vi "Module Init.vi"(8 "error in (no error)":errorcluster, 11 "Telemetry Server Module in":refnum<class "Telemetry Server Module.lvclass">) -> (0 "error out":errorcluster, 3 "Telemetry Server Module out":refnum<class "Telemetry Server Module.lvclass">)   [LabVIEW 2020, in "Volatus.lvlib" / "Telemetry Server Module.lvclass"]
uses:
  Telemetry Server Module.lvclass
  Telemetry Server Module.lvclass/Telemetry Server Module.ctl
  Module/Module.lvclass
  C:/dev/lv20CE/relink/lv-volatus/Volatus/Module/Module.lvclass
  C:/dev/lv20CE/relink/lv-volatus/Volatus/Telemetry Server Module/Telemetry Server Module.lvclass
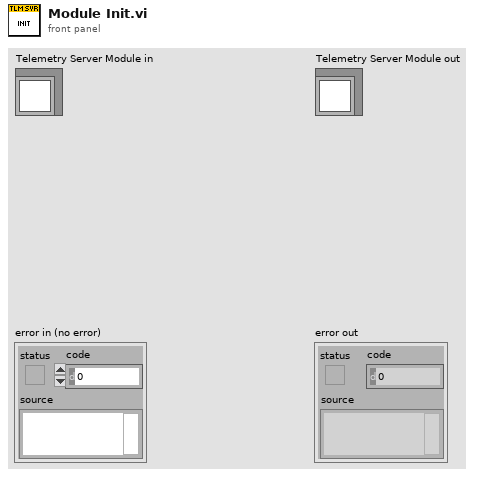
[diagram p1: front panel]
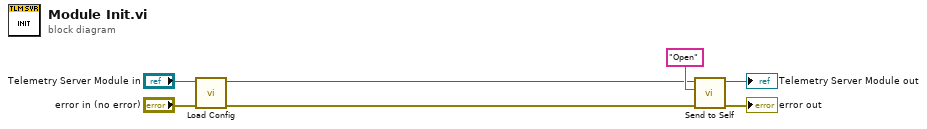
[diagram p0: block diagram]
diagram:
  n1 = call "Load Config.vi"("error in (no error)"="error in (no error)", "Telemetry Server Module in"="Telemetry Server Module in") -> ("error out"=w3:errorcluster, "Telemetry Server Module out"=w1:refnum<class "Telemetry Server Module.lvclass">)  [unwired: 8 in]
  n2 = call "Send to Self.vi"("error in (no error)"=w3, "Message ID"="Open", "Module in"=w1) -> ("error out"=→"error out":errorcluster, "Module out"=→"Telemetry Server Module out":refnum<class "Telemetry Server Module.lvclass">)  [unwired: 7 in]
